vi "HEWH Heat Elements.vi"(0 "VISA session":refnum<visa-resource-name>="MW100", 2 "Semiphore":T2, 5 "RS232 Data In":string[][](array[string]), 11 "Error In":errorcluster) -> (4 "dup VISA session":refnum<visa-resource-name>, 6 "POWER":T1, 15 "error out":errorcluster)   [LabVIEW 2009]
uses:
  PowerElements.ctl
  ChannelSettings.ctl
panel:
  out "Fan":bool
  out "Compressor":bool
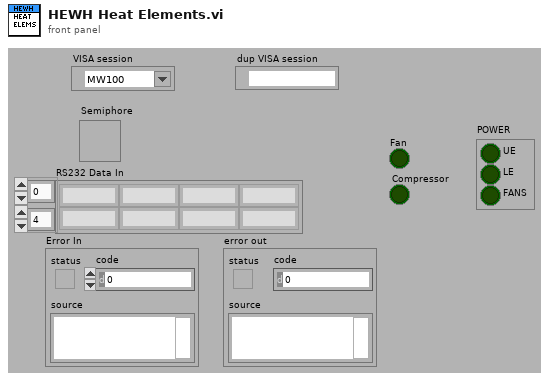
[diagram p1: front panel]
types:
  T1 = typedef "PowerElements.ctl" = cluster{"UE":bool, "LE":bool, "FANS":bool}
  T2 = typedef "Semaphore RefNum" = refnum<k1>
  T3 = typedef "ChannelSettings.ctl" = u32
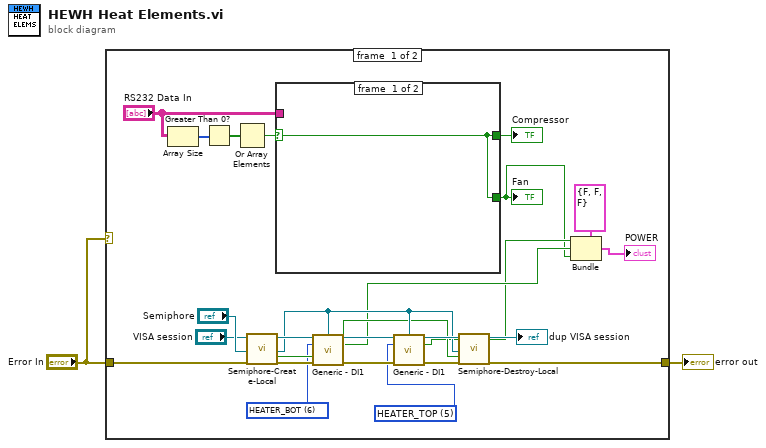
[diagram p0: block diagram]
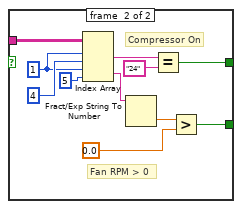
[diagram p2: hidden frame]
diagram:
  n1 = case shown="No Error" "Error In" {
    tunnel: "Error In" -> [w21 w38]
    tunnel: [w15 w38] -> w2
    frame #0 {
      w8 = T3 5 items=["4-20_OUT", "Pres_HI1", "Pres_HI2", "Pres_LOW", "Pres_PIN", "HEATER_TOP", "HEATER_BOT", "T_Shell", "FLOWMETER", "WATT_SENSE", "WH_TICK", "Tc_1", "Tc_2", "Tc_3", "Tc_4", "Tc_5", "Tc_6", "Tc_down", "T_Shell_2", "T_Shell_3", "T_Shell_4", "RTD_IN", "RTD_OUT", "RTD_AMB", "INTF_TEMPFLO", "INTF_READY", "INTF_START", "INTF_STOP", "DRM_LOW", "DRM_HIGH", "PWR_MAIN", "VLV_DUMP", "VLV_OUT", "VLV_IN", "WATT_HOURS", "FLOW(SAMPLE)", "GALLONS", "FLOW(GPM)"] ("Channel_Enum")
      w9 = T3 6 items=["4-20_OUT", "Pres_HI1", "Pres_HI2", "Pres_LOW", "Pres_PIN", "HEATER_TOP", "HEATER_BOT", "T_Shell", "FLOWMETER", "WATT_SENSE", "WH_TICK", "Tc_1", "Tc_2", "Tc_3", "Tc_4", "Tc_5", "Tc_6", "Tc_down", "T_Shell_2", "T_Shell_3", "T_Shell_4", "RTD_IN", "RTD_OUT", "RTD_AMB", "INTF_TEMPFLO", "INTF_READY", "INTF_START", "INTF_STOP", "DRM_LOW", "DRM_HIGH", "PWR_MAIN", "VLV_DUMP", "VLV_OUT", "VLV_IN", "WATT_HOURS", "FLOW(SAMPLE)", "GALLONS", "FLOW(GPM)"] ("Channel_Enum")
      n2 = Array Size(array="RS232 Data In") -> (size(s)=w24:i32[])
      n3 = Greater Than 0?(x=w24) -> (x > 0?=w23:bool[])
      n4 = Or Array Elements(Boolean array=w23) -> (logical OR=w22:bool)
      n5 = call "Semiphore-Create-Local.vi"("Semiphore"="Semiphore", "error in (no error)"=w21) -> ("semaphore"=w12:T2, "Local?"=w11:bool, "error out"=w18:errorcluster)  [unwired: 15 in]
      n6 = case shown="True" w22 {
        selector: w22 -> [w26 _]
        tunnel: [w26 w28] -> w10
        tunnel: "RS232 Data In" -> [_ w29]
        tunnel: [w26 w27] -> w3
        frame #0 {
        }
        frame #1 {
          w34 = 1 ("index (row)")
          # "Compressor On"
          # "Fan RPM > 0"
          n7 = Index Array(array=w29, index (row) #1=w34, index (col) #1=4 ("disabled index (col)"), index (row) #2=w34, index (col) #2=5 ("disabled index (col)")) -> (element #1=w36:string, element #2=w32:string)
          n8 = Fract/Exp String To Number(string=w32) -> (number=w31:dbl)  [unwired: 3 in, 1 out]
          n9 = Equal?(x=w36, y="24") -> (x = y?=w28:bool)
          n10 = Greater?(x=w31, y=0.0) -> (0:w27:bool)
        }
      }
      "Compressor" <- w10
      "Fan" <- w3
      n11 = call "Generic - DI1.vi"("VISA session"="VISA session", "Semiphore"=w12, "Channel_Enum"=w9, "Error In"=w18) -> ("dup VISA session"=w20:refnum<visa-resource-name>, "Value"=w5:bool, "error out"=w17:errorcluster)  [unwired: 9 in]
      n12 = call "Generic - DI1.vi"("VISA session"=w20, "Semiphore"=w12, "Channel_Enum"=w8, "Error In"=w17) -> ("dup VISA session"=→"dup VISA session":refnum<visa-resource-name>, "Value"=w4:bool, "error out"=w16:errorcluster)  [unwired: 9 in]
      n13 = call "Semiphore-Destroy-Local.vi"("Semiphore"=w12, "Local?"=w11, "error in (no error)"=w16) -> ("error out"=w15:errorcluster)  [unwired: 16 in]
      n14 = Bundle(cluster=T1 {"UE"=FALSE, "LE"=FALSE, "FANS"=FALSE} ("POWER 2"), "UE"=w4, "LE"=w5, "FANS"=w3) -> (→"POWER":T1)
    }
    frame #1 {
    }
  }
  "error out" <- w2
